vi "SCMP write init xml.vi"(8 "error in (no error)":errorcluster, 11 "FITS Header In":T1={"Wavelength (nm)"=530.15, "Exposure (s)"=0.05, "Tuning Delay (ms)"=1000.0, "Beam Type (-1/1)"=1.0, "Tuning Voltages"=[1.111, 2.222, 3.333, 4.444], "Observer"="observer", "Light Shapping Diffuser"=enum."In Beam", "Comment"="", "Data Type"=enum."HOLE", "Mod Cycles"=0, "SCD Calibration Optics"=enum."1 - Polarizer @0, I+Q", "SCD Emission Line Filter"=enum."1-557.6nm", "Cookbook"="", "COMP-S Calibration Wheel"=enum."Dark", "COMP-S Andover Filter Wheel"=enum."530.3nm/HWB 0.34nm (Fe XIV)", "FOV Rotation (deg)"=66.0, "Objective Lens Position (mm)"=0.0, "Occulter size"=0.0, "Time End"=timestamp(3382374145.421875 s since 1904-01-01), "Acc Exposure (s)"=0.0, "Time Stamp Array"=[], "Camera Serial Number"=[], "Camera Temp"=[], "Camera PI (mm)"=[], "Time Start"=timestamp(3382374145.421875 s since 1904-01-01), "Peripherals"={"ILX controler"=FALSE, "Zone temperatures"=FALSE, "Andor"=FALSE, "Andor 2"=FALSE, "PI Stages"=FALSE, "AISAS mechanisms"=FALSE, "AISAS Mech.lvclass"=refnum, "Zone temp ref"=variant, "FWs"=FALSE}, "FITS paths"=[], "Cameras"=enum."Andor", "load preset cbk"=FALSE, "periodic check count"=0, "COMP-S Calibration Wheel 2"=enum."Dark", "Calib"=enum."Dark", "Abso Aperture"=40.0, "Nominal Aperture"=196.0, "Pointer IP"="127.0.0.1"} {"Nominal Aperture" format="%.1f"; "Abso Aperture" format="%.1f"; "Camera PI (mm)" format="%_3g"; "Acc Exposure (s)" format="%^.3g"; "Occulter size" format="%.2f"; "Objective Lens Position (mm)" min=70.0 max=152.0 format="%.2f"; "FOV Rotation (deg)" format="%.1f"; "Exposure (s)" format="%^.3g"; "Wavelength (nm)" format="%_6g"}) -> (0 "error out":errorcluster, 3 "XML String":string)   [LabVIEW 2014]
uses:
  Controls/SCD - FITS Cluster.ctl
  AISAS/Mech/AISAS Mech.lvclass
  AISAS/Controls/Diffuser.ctl
  Controls/FITS Data type.ctl
  Controls/SCD - Calibration Optics Filter Wheel.ctl
  Controls/SCD - EDT - Emission Line Filter Wheel.ctl
  Controls/CoMP-S Controls/Polarization Optics Filter Wheel.ctl
  Controls/CoMP-S Controls/Emission Line Filter Wheel.ctl
  AISAS/Controls/focus.ctl
  Controls/peripherals.ctl
  Controls/Cameras select.ctl
  <vilib>/Utility/xml.llb/Write to XML File.vi
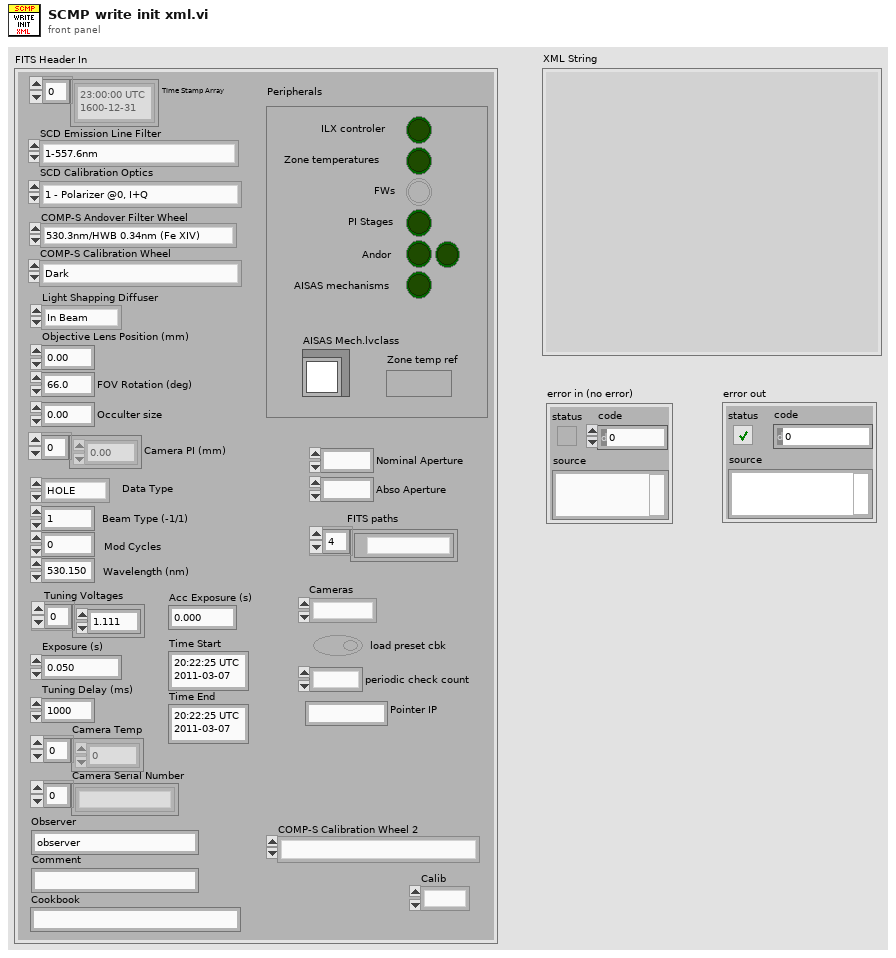
[diagram p1: front panel]
types:
  T1 = typedef "SCD - FITS Cluster.ctl" = cluster{"Wavelength (nm)":dbl, "Exposure (s)":dbl, "Tuning Delay (ms)":dbl, "Beam Type (-1/1)":dbl, "Tuning Voltages":dbl[], "Observer":string, "Light Shapping Diffuser":T2, "Comment":string, "Data Type":T3, "Mod Cycles":u16, "SCD Calibration Optics":T4, "SCD Emission Line Filter":T5, "Cookbook":string, "COMP-S Calibration Wheel":T6, "COMP-S Andover Filter Wheel":T7, "FOV Rotation (deg)":dbl, "Objective Lens Position (mm)":T8, "Occulter size":dbl, "Time End":timestamp, "Acc Exposure (s)":dbl, "Time Stamp Array":timestamp[], "Camera Serial Number":string[], "Camera Temp":dbl[], "Camera PI (mm)":dbl[], "Time Start":timestamp, "Peripherals":T9, "FITS paths":path[], "Cameras":T10, "load preset cbk":bool, "periodic check count":i32, "COMP-S Calibration Wheel 2":T6, "Calib":enum16{"Dark", "Flat"}, "Abso Aperture":dbl, "Nominal Aperture":dbl, "Pointer IP":string}
  T2 = typedef "Diffuser.ctl" = enum16{"Out of Beam", "In Beam"}
  T3 = typedef "FITS Data type.ctl" = enum16{"LIVE", "DARK", "FLAT", "CALI", "OBSE", "ABSO", "AURE", "TARG", "OBJE", "HOLE", "OREX", "THRO", "CHIP"}
  T4 = typedef "SCD - Calibration Optics Filter Wheel.ctl" = enum16{"1 - Polarizer @0, I+Q", "2 - Polarizer @90, I-Q", "3 - Polarizer @45, I+U", "4 - Polarizer @135, I-U", "5 - Polarizer @0, Retarder @45, I+V", "6 - Polarizer @0, Retarder @135, I-V", "7 - Dark", "8 - Clear", "9 - N/A"}
  T5 = typedef "SCD - EDT - Emission Line Filter Wheel.ctl" = enum16{"1-557.6nm", "2-587.6nm", "3-589.6nm", "4-630.2nm", "5-656.4nm", "6-849.8nm", "7-854.2nm", "8-866.2nm", "9-1083.0nm"}
  T6 = typedef "Polarization Optics Filter Wheel.ctl" = enum16{"Dark", "Clear", "Exchange Lens", "Polarizer @0, I+Q", "Polarizer @90, I-Q", "Polarizer @45, I+U", "Polarizer @135, I-U", "Polarizer @0, Retarder @45, I+V", "Polarizer @0, Retarder @135, I-V"}
  T7 = typedef "Emission Line Filter Wheel.ctl" = enum16{"530.3nm/HWB 0.34nm (Fe XIV)", "587.6nm/HBW 0.44nm (He I D3)", "637.5nm/HBW 0.53nm (Fe X)", "656.3nm/HBW 0.57nm (H-Alpha)", "789.2nm/HBW 0.85nm (Fe XI)", "854.2nm/HBW 1.01nm (Ca I)", "1074.7nm/HBW 2.34nm (Fe XIII)", "1079.8nm/HBW 1.64nm (Fe XIII)", "1083.0nm/HBW 1.66nm (He I)"}
  T8 = typedef "focus.ctl" = dbl
  T9 = typedef "peripherals.ctl" = cluster{"ILX controler":bool, "Zone temperatures":bool, "Andor":bool, "Andor 2":bool, "PI Stages":bool, "AISAS mechanisms":bool, "AISAS Mech.lvclass":refnum<class "AISAS Mech.lvclass">, "Zone temp ref":variant, "FWs":bool}
  T10 = typedef "Cameras select.ctl" = enum16{"Andor", "GDR"}
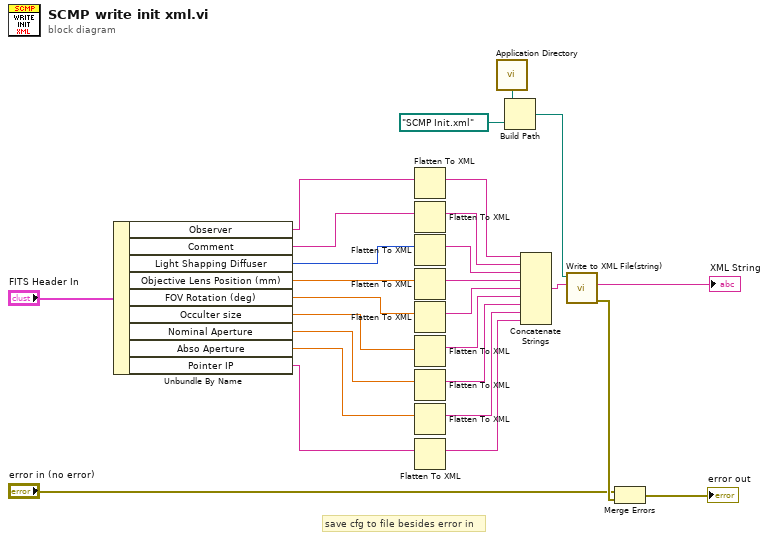
[diagram p0: block diagram]
diagram:
  # "save cfg to file besides error in"
  n1 = Unbundle By Name("FITS Header In") -> ("Observer"=w10:string, "Comment"=w9:string, "Light Shapping Diffuser"=w16:T2, "Objective Lens Position (mm)"=w15:T8, "FOV Rotation (deg)"=w14:dbl, "Occulter size"=w13:dbl, "Nominal Aperture"=w6:dbl, "Abso Aperture"=w5:dbl, "Pointer IP"=w2:string)
  n2 = Flatten To XML(anything=w10) -> (xml string=w7:string)
  n3 = Flatten To XML(anything=w9) -> (xml string=w8:string)
  n4 = Flatten To XML(anything=w16) -> (xml string=w20:string)
  n5 = Flatten To XML(anything=w15) -> (xml string=w22:string)
  n6 = Flatten To XML(anything=w14) -> (xml string=w23:string)
  n7 = Flatten To XML(anything=w13) -> (xml string=w21:string)
  n8 = Flatten To XML(anything=w6) -> (xml string=w4:string)
  n9 = Flatten To XML(anything=w5) -> (xml string=w3:string)
  n10 = Flatten To XML(anything=w2) -> (xml string=w1:string)
  n11 = call <vilib>:"Application Directory.vi"() -> ("Application Directory"=w18:path)
  n12 = Build Path(base path=w18, name or relative path=path "SCMP Init.xml" ("default name")) -> (appended path=w17:path)
  n13 = Concatenate Strings(w7, w8, w20, w22, w23, w21, w4, w3, w1) -> (w24:string)
  n14 = call-poly <vilib>:"Write to XML File(string).vi"("XML Input"=w24, "XML File Path"=w17) -> ("error out"=w12:errorcluster, "XML String"=→"XML String":string)  [unwired: 3 in, 5 out]
  n15 = Merge Errors("error in (no error)", w12) -> (→"error out":errorcluster)
